vi "Find VI in Project.vi"(8 "error in":errorcluster, 9 "VI Name":string, 10 "Non-Qualified VI Name":string, 11 "Project Items":refnum<vi>[](array[refnum])) -> (0 "error out":errorcluster, 2 "VI Found":bool)   [LabVIEW 2020]
doc: "Recursive VI used to search for the desired VI by name, Non-Qualified (as a project item) and Qualified (VI itself).\n\nRecursion is used to traverse the tree structure of the project."
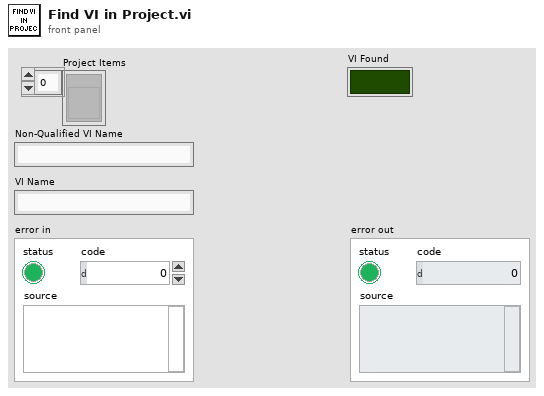
[diagram p1: front panel]
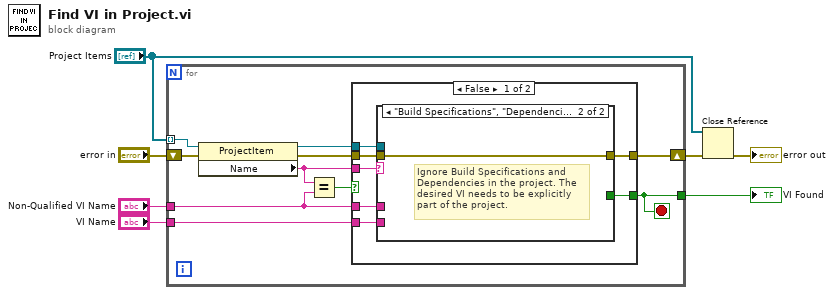
[diagram p0: block diagram]
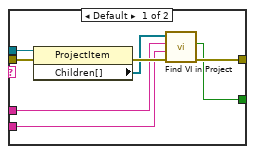
[diagram p2: hidden frame]
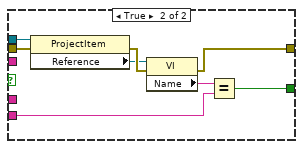
[diagram p3: hidden frame]
diagram:
  n1 = for {
    tunnel: "Project Items" -> [w14] mode=indexing
    tunnel: "VI Name" -> [w10]
    shift-right: [w15] -> w6
    shift-left: "error in" -> [w17]
    tunnel: "Non-Qualified VI Name" -> [w8]
    tunnel: [w9] -> w2
    stop <- w9 stop-if-true
    n2 = property class="ProjectItem"(reference=w14, error in=w17) -> (reference out=w13:refnum<vi>, error out=w16:errorcluster, "Name"=w12:string)
    n3 = Equal?(x=w12, y=w8) -> (x = y?=w11:bool)
    n4 = case shown="False" w11 {
      tunnel: w16 -> [w24 w41]
      tunnel: [w23 w39] -> w15
      tunnel: w13 -> [w22 w37]
      tunnel: w12 -> [w21 _]
      tunnel: w10 -> [w18 w35]
      tunnel: [w20 w34] -> w9
      tunnel: w8 -> [w19 _]
      frame False {
        n5 = case shown="\"Build Specifications\", \"Dependencies\"" w21 {
          tunnel: w24 -> [w32 w33]
          tunnel: [w30 w33] -> w23
          tunnel: w22 -> [w29 _]
          tunnel: [w28 _] -> w20
          tunnel: w19 -> [w26 _]
          tunnel: w18 -> [w27 _]
          frame Default {
            n6 = property class="ProjectItem"(reference=w29, error in=w32) -> (error out=w31:errorcluster, "Children[]"=w25:refnum<vi>[])  [unwired: 1 out]
            n7 = call "Find VI in Project.vi"("error in"=w31, "VI Name"=w27, "Non-Qualified VI Name"=w26, "Project Items"=w25) -> ("error out"=w30:errorcluster, "VI Found"=w28:bool)  [unwired: 6 in]
          }
          frame "Build Specifications", "Dependencies" {
            # "Ignore Build Specifications and Dependencies in the project. The desired VI needs to be explicitly part of the project."
          }
        }
      }
      frame True {
        n8 = property class="ProjectItem"(reference=w37, error in=w41) -> (error out=w40:errorcluster, "Reference"=w38:refnum<vi>)  [unwired: 1 out]
        n9 = property class="VI"(reference=w38, error in=w40) -> (error out=w39:errorcluster, "Name"=w36:string)  [unwired: 1 out]
        n10 = Equal?(x=w36, y=w35) -> (x = y?=w34:bool)
      }
    }
  }
  "VI Found" <- w2
  n11 = Close Reference(reference="Project Items", error in (no error)=w6) -> (error out=→"error out":errorcluster)
